vi "sub_checkPuzzleStatus.vi"(11 "puzzle (in)":string[][](array[string])) -> (2 "invalid item":string, 3 "status":enum16{"unsolved", "solved", "invalid state"}(ring))   [LabVIEW 2018]
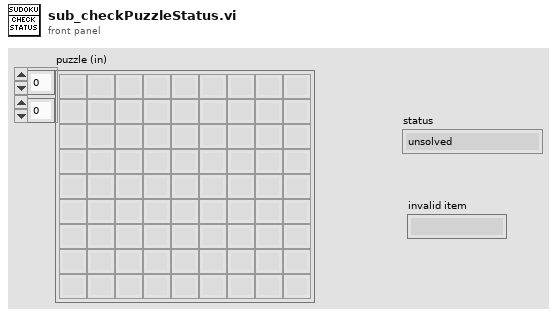
[diagram p1: front panel]
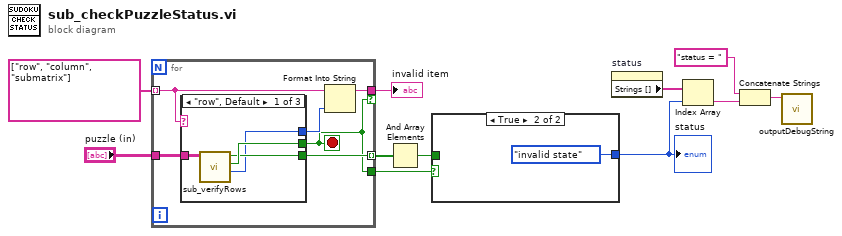
[diagram p0: block diagram]
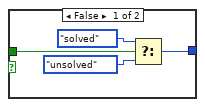
[diagram p2: hidden frame]
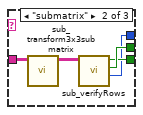
[diagram p3: hidden frame]
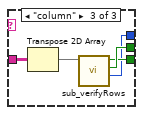
[diagram p4: hidden frame]
diagram:
  n1 = for {
    tunnel: "puzzle (in)" -> [w17]
    tunnel: string[] ["row", "column", "submatrix"] -> [w15] mode=indexing
    tunnel: [w16] -> w9 mode=indexing
    tunnel: [w12] -> w8
    tunnel: [w13] -> w6 if=w12
    stop <- w12 stop-if-true
    n2 = case shown="\"row\", Default" w15 {
      tunnel: w17 -> [w21 w23 w31]
      tunnel: [w20 w26 w30] -> w12
      tunnel: [w19 w25 w29] -> w16
      tunnel: [w18 w22 w27] -> w14
      frame "row", Default {
        n3 = call "sub_verifyRows.vi"("puzzle (in)"=w21) -> ("invalid row"=w18:i32, "invalid ?"=w20:bool, "solved ?"=w19:bool)  [unwired: 8 in]
      }
      frame "submatrix" {
        n4 = call "sub_transform3x3submatrix.vi"("puzzle (in)"=w23) -> ("transformed submatrix"=w24:string[][])  [unwired: 10 in]
        n5 = call "sub_verifyRows.vi"("puzzle (in)"=w24) -> ("invalid row"=w22:i32, "invalid ?"=w26:bool, "solved ?"=w25:bool)  [unwired: 8 in]
      }
      frame "column" {
        n6 = Transpose 2D Array(2D array=w31) -> (transposed array=w28:string[][])
        n7 = call "sub_verifyRows.vi"("puzzle (in)"=w28) -> ("invalid row"=w27:i32, "invalid ?"=w30:bool, "solved ?"=w29:bool)  [unwired: 8 in]
      }
    }
    n8 = Format Into String(initial string=w15, w14) -> (resulting string=w13:string)  [unwired: 2 in, 1 out]
  }
  "invalid item" <- w6
  n9 = And Array Elements(Boolean array=w9) -> (logical AND=w7:bool)
  n10 = case shown="True" w8 {
    tunnel: [w32 enum16{"unsolved", "solved", "invalid state"}."invalid state" ("status")] -> w4
    tunnel: w7 -> [w35 _]
    frame False {
      n11 = Select(t=enum16{"unsolved", "solved", "invalid state"}."solved", s=w35, f=enum16{"unsolved", "solved", "invalid state"}."unsolved" ("status")) -> (s? t:f=w32:enum16{"unsolved", "solved", "invalid state"})
    }
    frame True {
    }
  }
  "status" <- w4
  n12 = property on="status" class="Enum (strict)"() -> ("Strings []"=w5:string[])  [unwired: 2 in, 2 out]
  n13 = Index Array(array=w5, index=w4) -> (element=w2:string)
  n14 = Concatenate Strings("status = " ("string"), w2) -> (w1:string)
  n15 = call "outputDebugString.vi"("arg1"=w1) -> ()  [unwired: 11 in]
